vi "Measure.vi"(10 "t (seconds)":dbl, 11 "Sinusoid in":refnum<class "Sinusoid.lvclass">) -> (2 "y":dbl, 3 "Sinusoid out":refnum<class "Sinusoid.lvclass">)   [LabVIEW 2024, in "Sinusoid.lvclass"]
uses:
  Sinusoid.lvclass
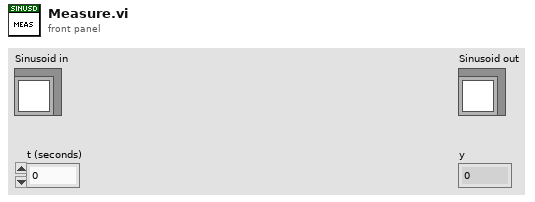
[diagram p1: front panel]
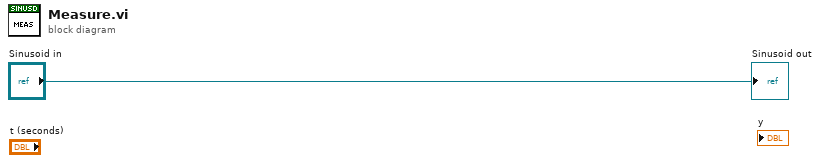
[diagram p0: block diagram]
diagram:
  "Sinusoid out" <- "Sinusoid in"
